vi "UpdateIntegration_PopUp.vi"(2 "error in (no error)":errorcluster, 4 "EpiWrapper in":refnum<class "EpiWrapper.lvclass">) -> (0 "error out":errorcluster, 1 "EpiWrapper out":refnum<class "EpiWrapper.lvclass">)   [LabVIEW 2012, in "EpiWrapper.lvclass"]
uses:
  EpiWrapper.lvclass
  EpiWrapper.lvclass/EpiWrapper.ctl
  Instruments.lvclass
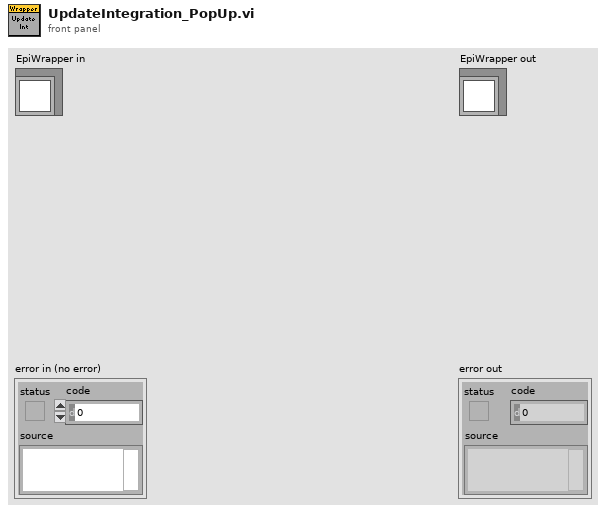
[diagram p1: front panel]
types:
  T1 = typedef "Config.ctl" = cluster{"IntTime":i32, "Samples":i32, "PowerMin":dbl, "KneeMin":dbl, "KneeMax":dbl, "Background Wl":dbl, "Settle Delay,ms":u32, "StationId":sgl}
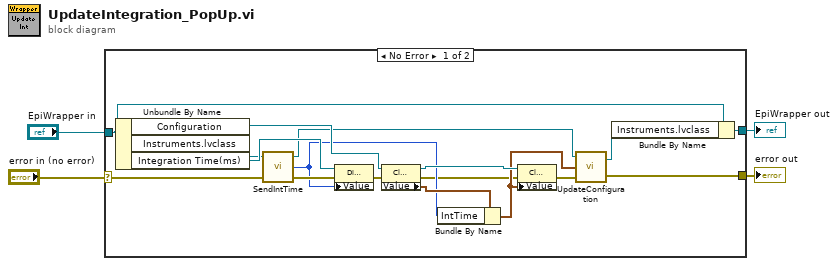
[diagram p0: block diagram]
diagram:
  n1 = case shown="No Error" "error in (no error)" {
    selector: "error in (no error)" -> [w10 w23]
    tunnel: [w21 w23] -> w3
    tunnel: [w18 w22] -> w1
    tunnel: "EpiWrapper in" -> [w20 w22]
    frame No Error {
      n2 = Unbundle By Name(w20) -> ("Configuration"=w16:refnum<vi>, "Instruments.lvclass"=w9:refnum<class "Instruments.lvclass">, "Integration Time(ms)"=w17:refnum<vi>)
      n3 = call-dynamic "SendIntTime.vi"("error in (no error)"=w10, "Instruments in"=w9) -> ("error out"=w8:errorcluster, "IntTime"=w7:i32, "Instruments out"=w5:refnum<class "Instruments.lvclass">)  [unwired: 1 in]
      n4 = property class="DigNum (strict)"(reference=w17, error in=w8, "Value"=w7) -> (error out=w15:errorcluster)  [unwired: 1 out]
      n5 = property class="Clust (strict)"(reference=w16, error in=w15) -> (reference out=w14:refnum<vi>, error out=w6:errorcluster, "Value"=w12:T1)
      n6 = Bundle By Name(cluster=w12, "IntTime"=w7) -> (w11:T1)
      n7 = property class="Clust (strict)"(reference=w14, error in=w6, "Value"=w11) -> (error out=w13:errorcluster)  [unwired: 1 out]
      n8 = call-dynamic "UpdateConfiguration.vi"("error in (no error)"=w13, "INSTR_PARAM.Config"=w11, "Instruments in"=w5) -> ("error out"=w21:errorcluster, "Instruments out"=w19:refnum<class "Instruments.lvclass">)
      n9 = Bundle By Name(cluster=w20, "Instruments.lvclass"=w19) -> (w18:refnum<class "EpiWrapper.lvclass">)
    }
    frame Error {
    }
  }
  "error out" <- w3
  "EpiWrapper out" <- w1
